vi "Read FlexLogger Data.vi"() -> ()   [LabVIEW 2024]
doc: "Demonstrates how to use network streams to pass data and commands between two running VIs. It displays waveform data that is received from the target VI and sends commands to update the frequency of the generated signal."
uses:
  <resource>/objmgr/ni.dex.rc
panel:
  out "Start Time":timestamp
  out "End Time":timestamp
  out "Connected to writer":bool
  in  "Writer IP Address":string="localhost"
  in  "stop":bool
  out "FlexLogger Data":waveform(dbl)[](graph)
  # "Overview: Demonstrates how to use Network Streams to read data from FlexLogger.\nRequirements: Windows\nInstructions:\n1. Add the StreamWriter plug-in in FlexLogger.\n2. Configure it using gear on right and map some channels using the channel picker and press OK.\n2. Run this VI.\n3. When done, click Stop to stop the VI."
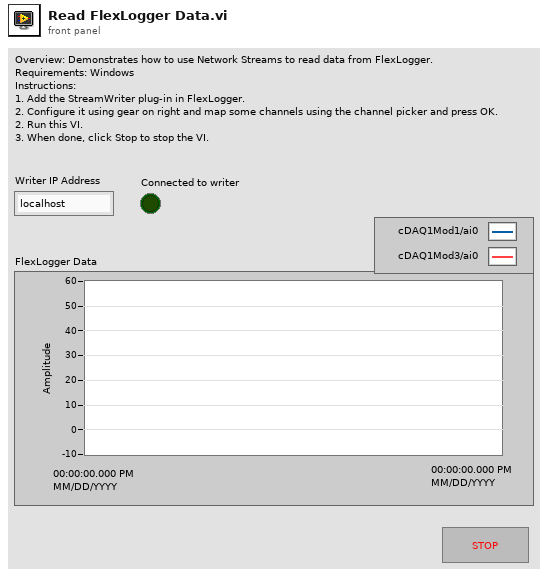
[diagram p1: front panel]
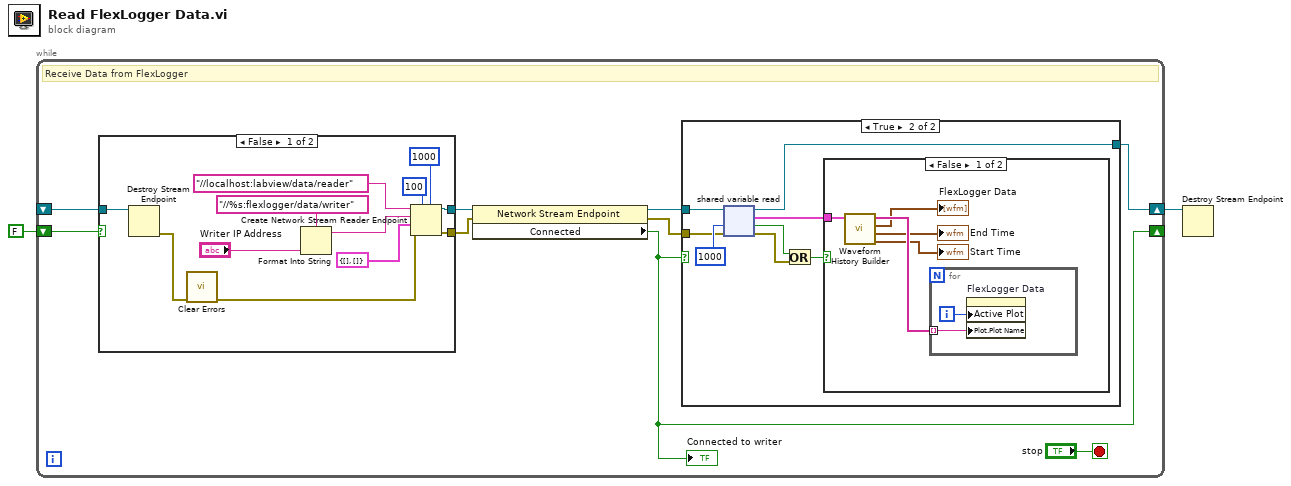
[diagram p0: block diagram]
diagram:
  n1 = while "Target->Host Data Reader" {
    shift-right: [w11] -> w2
    shift-left: _ -> [w9]
    shift-right: [w3] -> _
    shift-left: FALSE -> [w8]
    stop <- "stop" stop-if-true
    # "Receive Data from FlexLogger"
    n2 = case shown="False" w8 {
      tunnel: [w30 w40] -> w7
      tunnel: w9 -> [w39 w40]
      tunnel: [w28 _] -> w6
      frame False {
        n3 = Destroy Stream Endpoint(11:w39) -> (0:w38:errorcluster)  [unwired: 1 in]
        n4 = call <vilib>:"Clear Errors.vi"("error in (no error)"=w38) -> ("error out"=w31:errorcluster)  [unwired: 5 in, 1 out]
        n5 = Format Into String(format string="//%s:flexlogger/data/writer" ("reader url"), "Writer IP Address") -> (resulting string=w37:string)  [unwired: 2 in, 1 out]
        n6 = Create Network Stream Reader Endpoint(5:1000 ("timeout in ms (-1)"), 7:100 ("reader buffer size"), 8:w31, 9:cluster{waveform(dbl)[], string[]} {[], []}, 10:w37, 11:"//localhost:labview/data/reader" ("writer name")) -> (0:w28:errorcluster, 3:w30:refnum<k21>)  [unwired: 1 in]
      }
      frame True {
      }
    }
    n7 = property class="Network Stream Endpoint"(reference=w7, error in=w6) -> (reference out=w5:refnum<k21>, error out=w4:errorcluster, "Connected"=w3:bool)
    "Connected to writer" <- w3
    n8 = case shown="True" w3 {
      tunnel: [w12 w17] -> w11
      tunnel: w5 -> [w12 w14]
      tunnel: w4 -> [_ w13]
      frame False {
      }
      frame True {
        n9 = shared-variable-read(w14, w13, 1000 ("timeout ms")) -> (w17:refnum<k21>, w16:errorcluster, w19:bool, w20:cluster{waveform(dbl)[], string[]})
        n10 = Or(x=w19, y=w16) -> (x .or. y?=w18:bool)
        n11 = case shown="False" w18 {
          tunnel: w20 -> [w25 _]
          frame False {
            n12 = call "Waveform History Builder.vi"("Data Read"=w25) -> ("Min Time"=→"Start Time":timestamp, "Max Time"=→"End Time":timestamp, "Waveforms"=→"FlexLogger Data":waveform(dbl)[], "Channel Names"=w24:string[])  [unwired: 7 in]
            n13 = for {
              tunnel: w24 -> [w27] mode=indexing
              i -> [w26]
              n14 = property on="FlexLogger Data" class="WFGraph (strict)"("Active Plot"=w26, "Plot.Plot Name"=w27) -> ()  [unwired: 2 in, 2 out]
            }
          }
          frame True {
          }
        }
      }
    }
  }
  n15 = Destroy Stream Endpoint(11:w2) -> ()  [unwired: 1 in, 1 out]
